vi "CreateLogHeader.vi"(10 "Names":string[][](array[string]), 11 "DUT Count":u32) -> (3 "Column Headers":string)   [LabVIEW 2012]
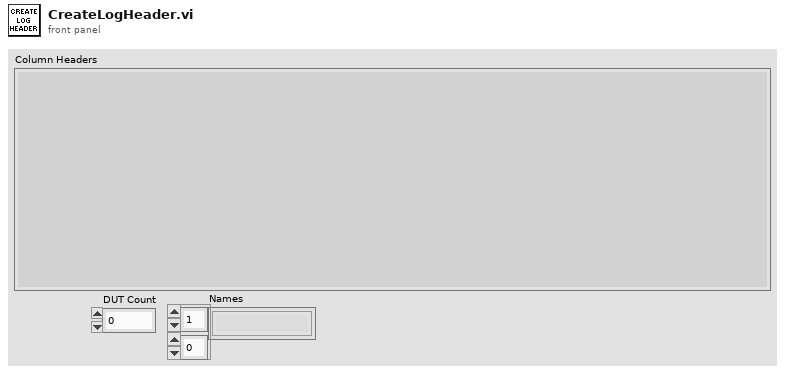
[diagram p1: front panel]
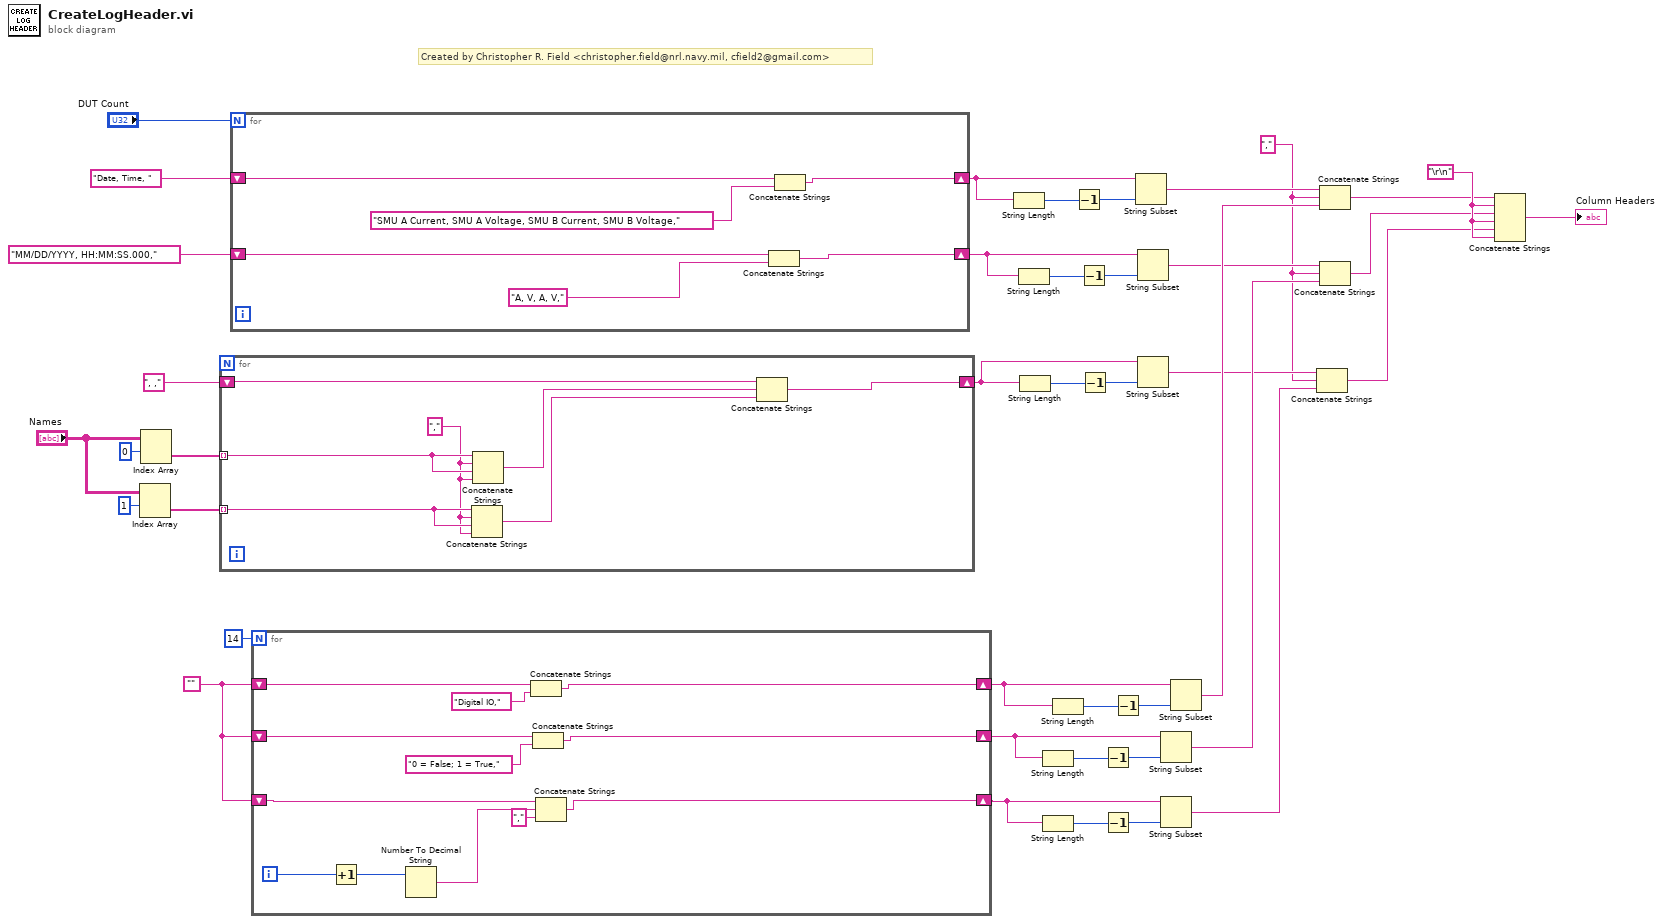
[diagram p0: block diagram]
diagram:
  w5 = ","
  w20 = ""
  w27 = "\r\n"
  # "Created by Christopher R. Field <christopher.field@nrl.navy.mil, cfield2@gmail.com>"
  n1 = Index Array(array="Names", index (row)=1) -> (element=w23:string[])  [unwired: 1 in]
  n2 = Index Array(array="Names", index (row)=0) -> (element=w24:string[])  [unwired: 1 in]
  n3 = for {
    shift-right: [w46] -> w22
    shift-left: ", ," -> [w45]
    tunnel: w24 -> [w44] mode=indexing
    tunnel: w23 -> [w43] mode=indexing
    w42 = "," ("string")
    n4 = Concatenate Strings(w43, w42, w43, w42) -> (w48:string)
    n5 = Concatenate Strings(w44, w42, w44, w42) -> (w47:string)
    n6 = Concatenate Strings(w45, w47, w48) -> (w46:string)
  }
  n7 = for {
    N: "DUT Count" -> [_]
    shift-right: [w53] -> w34
    shift-left: "Date, Time, " -> [w54]
    shift-right: [w50] -> w30
    shift-left: "MM/DD/YYYY, HH:MM:SS.000," -> [w51]
    n8 = Concatenate Strings(w51, "A, V, A, V," ("string")) -> (w50:string)
    n9 = Concatenate Strings(w54, "SMU A Current, SMU A Voltage, SMU B Current, SMU B Voltage,") -> (w53:string)
  }
  n10 = for {
    N: 14 -> [_]
    shift-right: [w64] -> w17
    shift-left: w20 -> [w66]
    shift-right: [w61] -> w14
    shift-left: w20 -> [w63]
    shift-right: [w56] -> w11
    shift-left: w20 -> [w59]
    i -> [w60]
    n11 = Increment(x=w60) -> (x+1=w58:i32)
    n12 = Number To Decimal String(number=w58) -> (decimal integer string=w57:string)  [unwired: 1 in]
    n13 = Concatenate Strings(w66, "Digital IO,") -> (w64:string)
    n14 = Concatenate Strings(w63, "0 = False; 1 = True,") -> (w61:string)
    n15 = Concatenate Strings(w59, w57, "," ("string")) -> (w56:string)
  }
  n16 = String Length(string=w34) -> (length=w35:i32)
  n17 = String Length(string=w30) -> (length=w32:i32)
  n18 = String Length(string=w22) -> (length=w29:i32)
  n19 = String Length(string=w14) -> (length=w16:i32)
  n20 = String Length(string=w11) -> (length=w13:i32)
  n21 = String Length(string=w17) -> (length=w19:i32)
  n22 = Decrement(x=w35) -> (x-1=w33:i32)
  n23 = Decrement(x=w32) -> (x-1=w31:i32)
  n24 = Decrement(x=w29) -> (x-1=w28:i32)
  n25 = Decrement(x=w16) -> (x-1=w15:i32)
  n26 = Decrement(x=w13) -> (x-1=w12:i32)
  n27 = Decrement(x=w19) -> (x-1=w18:i32)
  n28 = String Subset(string=w34, length (rest)=w33) -> (substring=w10:string)  [unwired: 1 in]
  n29 = String Subset(string=w30, length (rest)=w31) -> (substring=w8:string)  [unwired: 1 in]
  n30 = String Subset(string=w22, length (rest)=w28) -> (substring=w6:string)  [unwired: 1 in]
  n31 = String Subset(string=w14, length (rest)=w15) -> (substring=w7:string)  [unwired: 1 in]
  n32 = String Subset(string=w11, length (rest)=w12) -> (substring=w4:string)  [unwired: 1 in]
  n33 = String Subset(string=w17, length (rest)=w18) -> (substring=w9:string)  [unwired: 1 in]
  n34 = Concatenate Strings(w6, w5, w4) -> (w1:string)
  n35 = Concatenate Strings(w10, w5, w9) -> (w3:string)
  n36 = Concatenate Strings(w8, w5, w7) -> (w2:string)
  n37 = Concatenate Strings(w3, w27, w2, w27, w1, w27) -> (→"Column Headers":string)
